vi "example.vi"() -> ()   [LabVIEW 2023]
panel:
  out "Operating \nChannel(s)":bool[][](array[boolean])
  out "Array":i32[][](array[numeric])
  out "x":i32
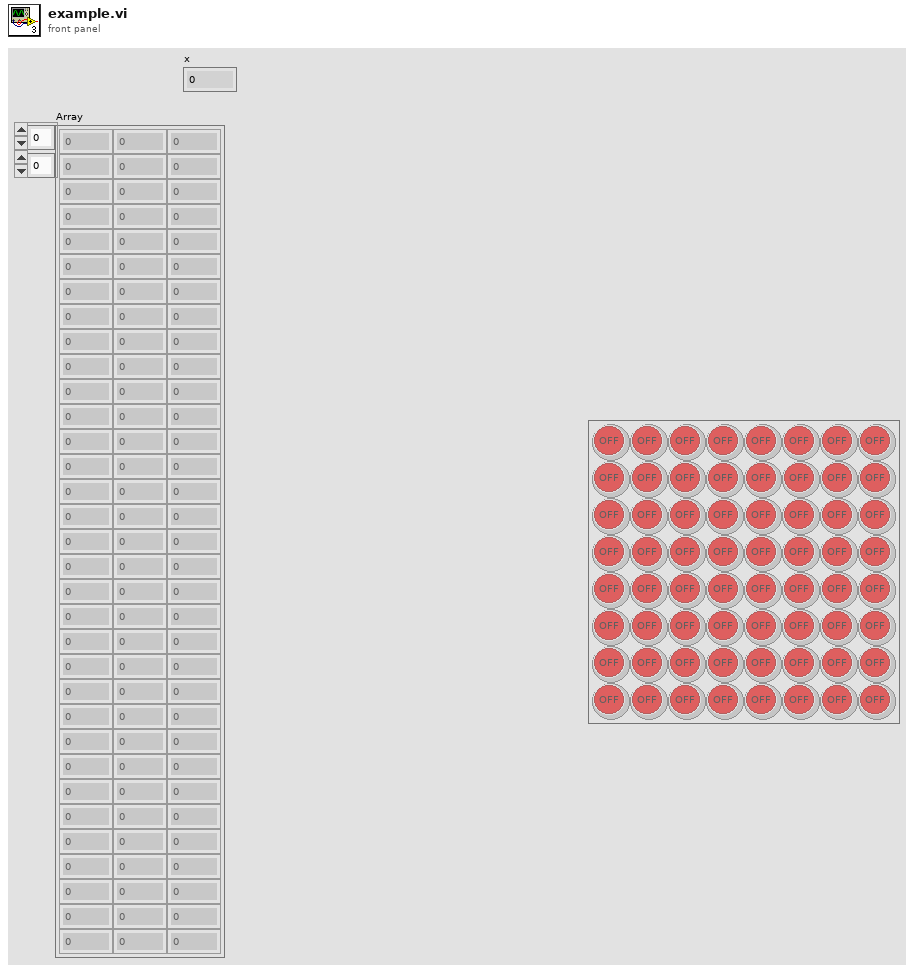
[diagram p1: front panel]
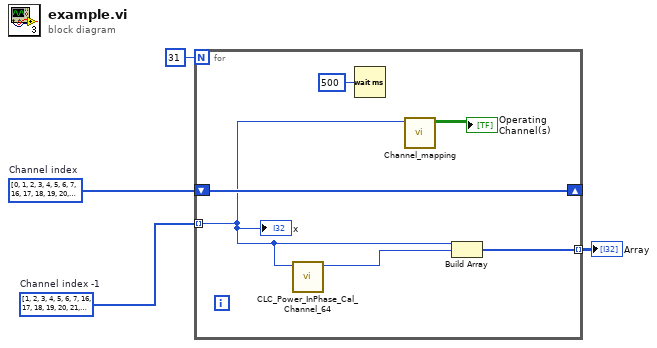
[diagram p0: block diagram]
diagram:
  w3 = i32[] [1, 2, 3, 4, 5, 6, 7, 16, 17, 18, 19, 20, 21, 22, 23, 32, 33, 34, 35, 36, 37, 38, 39, 48, 49, 50, 51, 52, 53, 54, 55]  # Channel index -1
  w2 = i32[] [0, 1, 2, 3, 4, 5, 6, 7, 16, 17, 18, 19, 20, 21, 22, 23, 32, 33, 34, 35, 36, 37, 38, 39, 48, 49, 50, 51, 52, 53, 54, 55]  # Channel index
  n1 = for {
    N: 31 -> [_]
    tunnel: w3 -> [w6] mode=indexing
    shift-right: [w9] -> _
    shift-left: w2 -> [w9]
    tunnel: [w8] -> w1 mode=indexing
    n2 = call "CLC_Power_InPhase_Cal_Channel_64.vi"("Channel IN"=w6) -> ("Ref_Channel"=w7:i32)  [unwired: 8 in, 2 out]
    n3 = Wait (ms)(milliseconds to wait=u32 500) -> ()  [unwired: 1 out]
    n4 = call "Channel_mapping.vi"("Channel IN"=w6) -> ("Operating \nChannel(s)"=→"Operating \nChannel(s)":bool[][])  [unwired: 10 in]
    n5 = Build Array(w6, w7) -> (w8:i32[])
    "x" <- w6
  }
  "Array" <- w1
